vi "_VI Tree.vi"   [LabVIEW 2018, in "labview_json.lvlib"]
uses:
  labview_json.lvlib
  Element Type.ctl
  Element.ctl
  c5bf3846-086a-4bf1-8521-c9c3fd3e4c1a.vi
  JSON Action.ctl
panel:
  # "SEE DIAGRAM\nFOR VI Tree"
types:
  T1 = typedef "labview_json.lvlib/JSON Action.ctl" = enum8{"Get or Create", "Get", "Set"}
  T2 = typedef "labview_json.lvlib/Element.ctl" = cluster{"Key":string, "Type":T3, "Value":variant}
  T3 = typedef "labview_json.lvlib/Element Type.ctl" = enum8{"NULL", "BOOL", "INT", "UINT", "FLOAT", "STRING", "ARRAY", "OBJECT", "SKIP"}
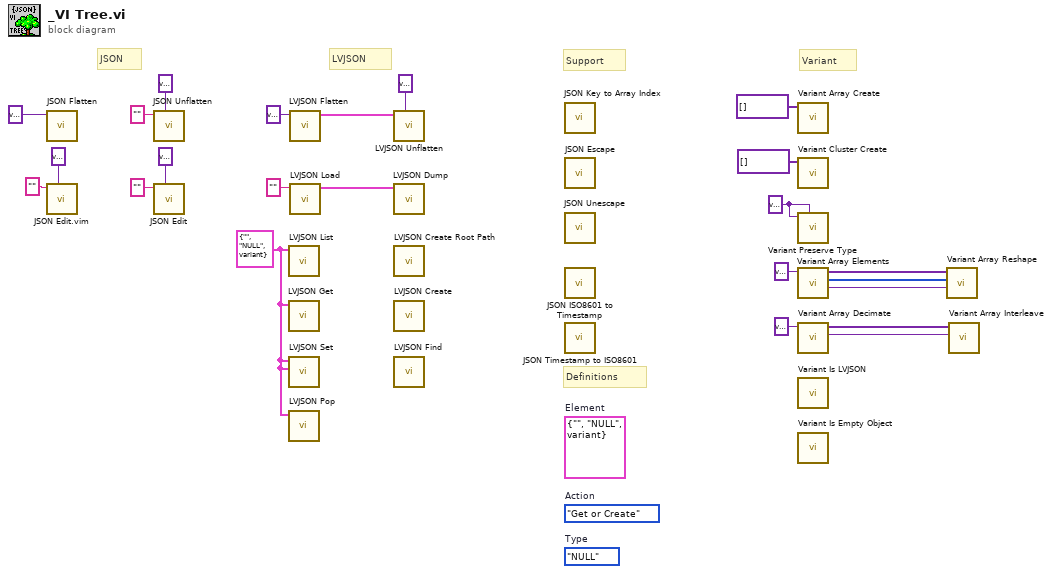
[diagram p0: block diagram]
diagram:
  (unwired) JSON_Action."Get or Create"  # Action
  (unwired) T2 {"Key"="", "Type"=enum."NULL", "Value"=variant}  # Element
  (unwired) Element_Type."NULL"  # Type
  w6 = T2 {"Key"="", "Type"=enum."NULL", "Value"=variant} ("Root Element in")
  w21 = variant ("Variant in")
  # "Definitions"
  # "Variant"
  # "LVJSON"
  # "Support"
  # "JSON"
  n1 = call "JSON Flatten.vi"("Variant in"=variant) -> ()  [unwired: 9 in, 2 out]
  n2 = call "JSON Edit.vim"("Variant in"=variant, "JSON in"="") -> ()  [unwired: 6 in, 4 out]
  n3 = call "JSON Unflatten.vi"("Variant Type"=variant, "JSON in"="") -> ()  [unwired: 7 in, 3 out]
  n4 = call "JSON Edit.vi"("Variant in"=variant, "JSON in"="") -> ()  [unwired: 6 in, 4 out]
  n5 = call "LVJSON List.vi"("Root Element in"=w6) -> ()  [unwired: 7 in, 4 out]
  n6 = call "LVJSON Get.vi"("Root Element in"=w6) -> ()  [unwired: 7 in, 4 out]
  n7 = call "LVJSON Set.vi"("Root Element to Merge"=w6, "Root Element in"=w6) -> ()  [unwired: 7 in, 3 out]
  n8 = call "LVJSON Pop.vi"("Root Element in"=w6) -> ()  [unwired: 7 in, 4 out]
  n9 = call "LVJSON Flatten.vi"("Variant in"=variant) -> ("Root Element out"=w10:T2)  [unwired: 9 in, 1 out]
  n10 = call "LVJSON Load.vi"("JSON in"="") -> ("Root Element out"=w11:T2)  [unwired: 8 in, 2 out]
  n11 = call "LVJSON Unflatten.vi"("Variant Type"=variant, "Root Element in"=w10) -> ()  [unwired: 6 in, 4 out]
  n12 = call "LVJSON Dump.vi"("Root Element in"=w11) -> ()  [unwired: 8 in, 3 out]
  n13 = call "LVJSON Create Root Path.vi"() -> ()  [unwired: 10 in, 2 out]
  n14 = call "LVJSON Create.vi"() -> ()  [unwired: 11 in, 1 out]
  n15 = call "LVJSON Find.vi"() -> ()  [unwired: 10 in, 2 out]
  n16 = call "JSON Key to Array Index.vi"() -> ()  [unwired: 9 in, 3 out]
  n17 = call "JSON Escape.vi"() -> ()  [unwired: 9 in, 3 out]
  n18 = call "JSON Unescape.vi"() -> ()  [unwired: 9 in, 3 out]
  n19 = call "JSON ISO8601 to Timestamp.vi"() -> ()  [unwired: 11 in, 1 out]
  n20 = call "JSON Timestamp to ISO8601.vi"() -> ()  [unwired: 11 in, 1 out]
  n21 = call "Variant Array Create.vi"("Elements"=variant[] []) -> ()  [unwired: 9 in, 2 out]
  n22 = call "Variant Cluster Create.vi"("Elements"=variant[] []) -> ()  [unwired: 9 in, 2 out]
  n23 = call "Variant Preserve Type.vi"("Variant Type"=w21, "Variant in"=w21) -> ()  [unwired: 8 in, 2 out]
  n24 = call "Variant Array Elements.vi"("N Dim Array"=variant) -> ("Element Type"=w16:variant, "Sizes"=w17:i32[], "Elements"=w18:variant[])  [unwired: 7 in, 1 out]
  n25 = call "Variant Array Decimate.vi"("N Dim Array"=variant) -> ("Element Type"=w13:variant, "Array of Variant Arrays"=w14:variant[])  [unwired: 7 in, 2 out]
  n26 = call "Variant Is LVJSON.vi"() -> ()  [unwired: 1 in, 1 out]
  n27 = call "Variant Is Empty Object.vi"() -> ()  [unwired: 1 in, 1 out]
  n28 = call "Variant Array Reshape.vi"("Default Element Type"=w16, "Sizes"=w17, "Elements"=w18) -> ()  [unwired: 7 in, 2 out]
  n29 = call "Variant Array Interleave.vi"("Default Element Type"=w13, "Array of Variant Arrays"=w14) -> ()  [unwired: 8 in, 2 out]
